vi "Process.vi"(8 "error in":errorcluster, 11 "Plugin in":refnum<class "StreamWriter.lvclass">) -> (0 "error out":errorcluster, 3 "Plugin out":refnum<class "StreamWriter.lvclass">)   [LabVIEW 2024, in "StreamWriter.lvlib" / "StreamWriter.lvclass"]
uses:
  StreamWriter.lvclass
  StreamWriter.lvclass/StreamWriter.ctl
  <resource>/objmgr/ni.dex.rc
  <vilib>/FlexLogger/SDK/PluginSDK.lvlibp/PEFClasses/SDK/Plugin/Plugin.lvclass
  C:/Program Files/National Instruments/LabVIEW 2024/vi.lib/FlexLogger/SDK/PluginSDK.lvlibp/PEFClasses/SDK/Plugin/Plugin.lvclass
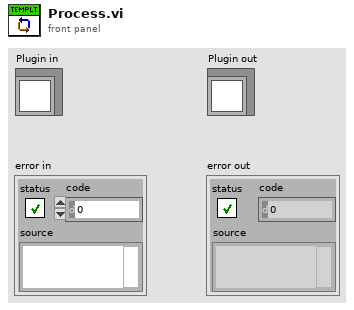
[diagram p1: front panel]
types:
  T1 = typedef "StreamWriter.lvlib/StreamWriter.lvclass/StreamWriter Parameters.ctl" = cluster{"Timeout":i32, "Buffer Size":i32, "Writer Endpoint":refnum<k21>}
  T2 = cluster{"Data":waveform(dbl)[], "Stream Names":string[]}
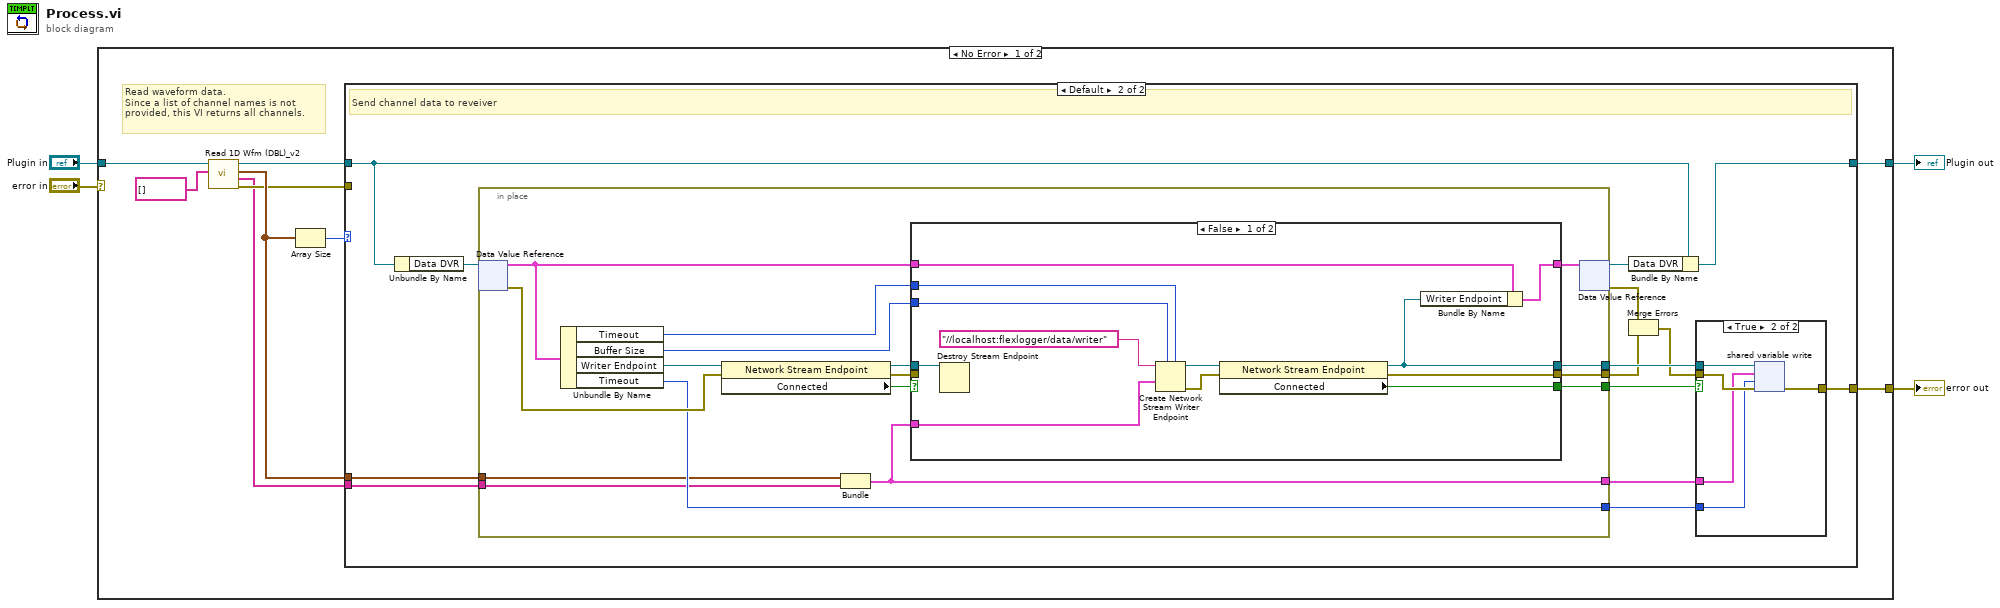
[diagram p0: block diagram]
diagram:
  n1 = case shown="No Error" "error in" {
    selector: "error in" -> [_ w67]
    tunnel: [w6 w68] -> w1
    tunnel: "Plugin in" -> [w7 w68]
    tunnel: [w5 w67] -> w2
    frame No Error {
      # "Read waveform data.\nSince a list of channel names is not provided, this VI returns all channels."
      n2 = call <vilib>:"Read 1D Wfm (DBL)_v2.vi"("Unique Identifers (empty = all)"=string[] [] ("Unique Channel Identifers (empty = all)"), "Plugin in"=w7) -> ("error out"=w10:errorcluster, "Stream Names"=w8:string[], "Data"=w13:waveform(dbl)[], "Plugin out"=w11:refnum<class "StreamWriter.lvclass">)  [unwired: 6 in]
      n3 = Array Size(array=w13) -> (size(s)=w12:i32)
      n4 = case shown="Default" w12 {
        tunnel: w13 -> [_ w18]
        tunnel: [w14 w29] -> w5
        tunnel: [w15 w22] -> w6
        tunnel: w11 -> [w15 w24]
        tunnel: w10 -> [w14 _]
        tunnel: w8 -> [_ w17]
        frame 0 {
          # "No channels sending data to the plugin"
        }
        frame Default {
          # "Send channel data to reveiver"
          n5 = Unbundle By Name(w24) -> ("Data DVR"=w26:refnum<data-value>)
          n6 = in-place {
            in-place-border: [w42] -> w21
            in-place-border: [w41] -> w28
            in-place-border: [w40] -> w27
            in-place-border: [w33] -> w19
            in-place-border: w18 -> [w32]
            in-place-border: w17 -> [w31]
            in-place-border: [w30] -> w16
            n7 = in-place-dvr #1(w26) -> (w36:T1, w34:errorcluster)
            n8 = Unbundle By Name(w36) -> ("Timeout"=w37:i32, "Buffer Size"=w38:i32, "Writer Endpoint"=w39:refnum<k21>, "Timeout"=w33:i32)
            n9 = property class="Network Stream Endpoint"(reference=w39, error in=w34) -> (reference out=w43:refnum<k21>, error out=w45:errorcluster, "Connected"=w44:bool)
            n10 = Bundle("Data"=w32, "Stream Names"=w31) -> (w30:T2)  [unwired: 1 in]
            n11 = case shown="False" w44 {
              selector: w44 -> [_ w59]
              tunnel: [w57 w58] -> w35
              tunnel: [w56 w60] -> w42
              tunnel: [w47 w61] -> w41
              tunnel: w43 -> [w55 w61]
              tunnel: [w54 w59] -> w40
              tunnel: w45 -> [_ w60]
              tunnel: w38 -> [w51 _]
              tunnel: w37 -> [w50 _]
              tunnel: w36 -> [w49 w58]
              tunnel: w30 -> [w48 _]
              frame False {
                n12 = Destroy Stream Endpoint(11:w55) -> ()  [unwired: 1 in, 1 out]
                n13 = Create Network Stream Writer Endpoint(5:w50, 7:w51, 9:w48, 11:"//localhost:flexlogger/data/writer" ("reader url")) -> (0:w52:errorcluster, 3:w53:refnum<k21>)  [unwired: 3 in]
                n14 = property class="Network Stream Endpoint"(reference=w53, error in=w52) -> (reference out=w47:refnum<k21>, error out=w56:errorcluster, "Connected"=w54:bool)
                n15 = Bundle By Name(cluster=w49, "Writer Endpoint"=w47) -> (w57:T1)
              }
              frame True {
              }
            }
            n16 = in-place-dvr #1(w35) -> (w23:refnum<data-value>, w25:errorcluster)
          }
          n17 = Bundle By Name(cluster=w24, "Data DVR"=w23) -> (w22:refnum<class "StreamWriter.lvclass">)
          n18 = Merge Errors(w25, w21) -> (w20:errorcluster)
          n19 = case shown="True" w27 {
            tunnel: w28 -> [_ w66]
            tunnel: w20 -> [_ w65]
            tunnel: [_ w64] -> w29
            tunnel: w16 -> [_ w63]
            tunnel: w19 -> [_ w62]
            frame False {
            }
            frame True {
              n20 = shared-variable-write(w66, w65, w63, w62) -> (w64:errorcluster)  [unwired: 2 out]
            }
          }
        }
      }
    }
    frame Error {
    }
  }
  "error out" <- w2
  "Plugin out" <- w1
